vi "SL_ReadData.vi"(11 "Tag":T2) -> (1 "type":string, 2 "value":string)   [LabVIEW 2019]
uses:
  SL_Control.ctl
panel:
  out "Value Read":string
  out "Number Read":dbl
  out "Comm":T1
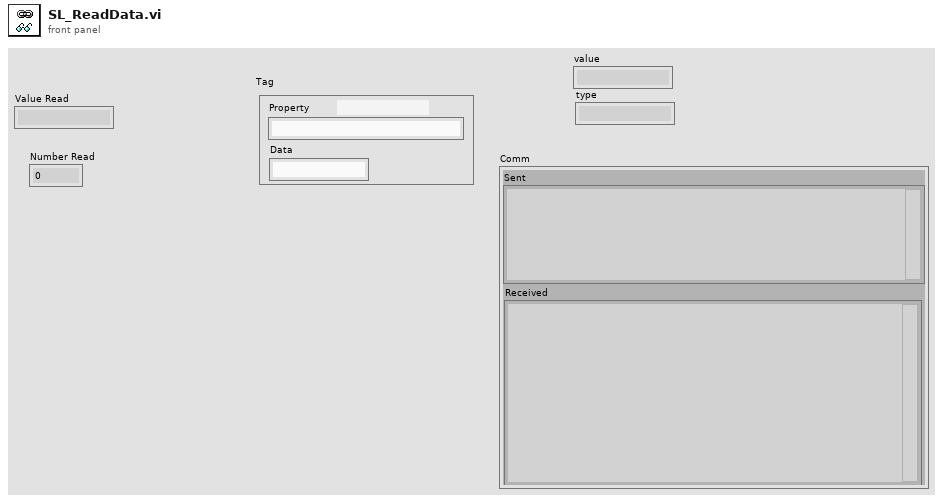
[diagram p1: front panel]
types:
  T1 = cluster{"url":string, "sent headers":string, "sent body":string, "headers":string, "body":string, "Sent":string, "Received":string}
  T2 = typedef "SL_Control.ctl" = cluster{"Property":string, "Type":string, "Data":string}
  T3 = enum16{"GET", "PUT", "POST", "MultiPOST", "DELETE"}
  T4 = cluster{"current":cluster{"timestamp":string, "value":cluster{"type":string, "value":string}}}
  T5 = cluster{"Name":string, "BaseURL":string, "AppKey":string, "Headers":string[], "Timeout":i32}
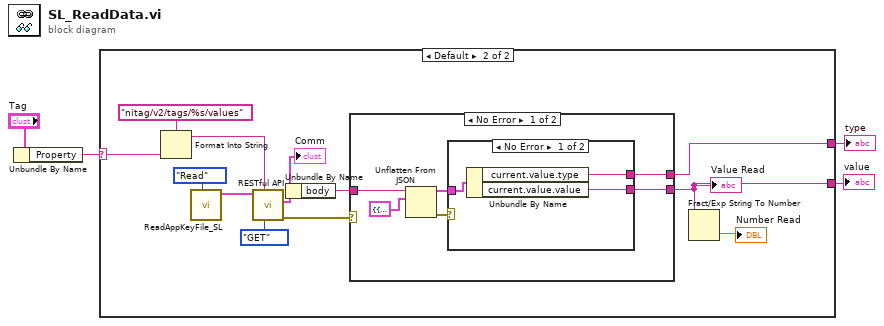
[diagram p0: block diagram]
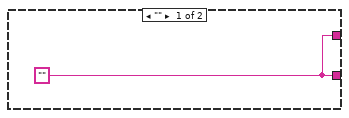
[diagram p2: hidden frame]
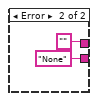
[diagram p3: hidden frame]
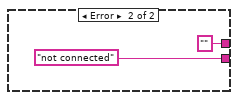
[diagram p4: hidden frame]
diagram:
  n1 = Unbundle By Name("Tag") -> ("Property"=w2:string)
  n2 = case shown="Default" w2 {
    selector: w2 -> [_ w12]
    tunnel: [w5 w7] -> w3
    tunnel: [w5 w6] -> w1
    frame "" {
      w5 = "" ("body")
    }
    frame Default {
      n3 = Format Into String(format string="nitag/v2/tags/%s/values" ("url"), w12) -> (resulting string=w11:string)  [unwired: 2 in, 1 out]
      n4 = call "ReadAppKeyFile_SL.vi"("Task"=enum16{"Read", "Write"}."Read") -> ("Device Out"=w17:T5)  [unwired: 8 in, 2 out]
      n5 = call "RESTful API.vi"("Method"=T3."GET", "url"=w11, "Device In"=w17) -> ("error out"=w8:errorcluster, "Comm"=w10:T1)  [unwired: 6 in, 1 out]
      "Comm" <- w10
      n6 = Unbundle By Name(w10) -> ("body"=w9:string)
      n7 = case shown="No Error" w8 {
        tunnel: [w19 "not connected" ("value")] -> w7
        tunnel: w9 -> [w20 _]
        tunnel: [w18 "" ("type")] -> w6
        frame No Error {
          n8 = Unflatten From JSON(JSON string=w20, type and defaults=T4 {"current"={"timestamp"="", "value"={"type"="", "value"=""}}}) -> (value=w21:T4, error out=w22:errorcluster)  [unwired: 5 in]
          n9 = case shown="No Error" w22 {
            tunnel: w21 -> [w26 _]
            tunnel: [w25 "None" ("value")] -> w19
            tunnel: [w24 "" ("type")] -> w18
            frame No Error {
              n10 = Unbundle By Name(w26) -> ("current.value.type"=w24:string, "current.value.value"=w25:string)
            }
            frame Error {
            }
          }
        }
        frame Error {
        }
      }
      "Value Read" <- w7
      n11 = Fract/Exp String To Number(string=w7) -> (number=→"Number Read":dbl)  [unwired: 3 in, 1 out]
    }
  }
  "value" <- w3
  "type" <- w1
